vi "park.vi"() -> ()   [LabVIEW 2015]
uses:
  <vilib>/Analysis/baseanly.llb/Mean (DBL).vi
  <vilib>/Analysis/NI_AALBase.lvlib
panel:
  out "SGL error max":dbl
  out "SGL error mean":dbl format="%0.2f"
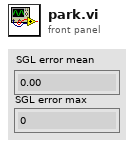
[diagram p1: front panel]
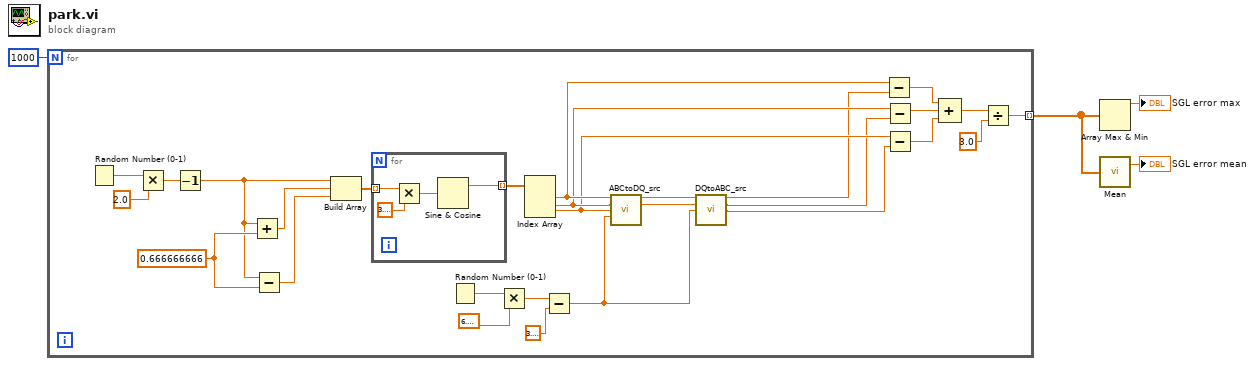
[diagram p0: block diagram]
diagram:
  n1 = for {
    N: 1000 -> [_]
    tunnel: [w19] -> w4 mode=indexing
    w30 = 0.666666666
    n2 = Random Number (0-1)() -> (number: 0 to 1=w18:dbl)
    n3 = Multiply(x=w18, y=2.0) -> (x*y=w31:dbl)
    n4 = Decrement(x=w31) -> (x-1=w25:dbl)
    n5 = Add(x=w25, y=w30) -> (x+y=w26:dbl)
    n6 = Subtract(x=w25, y=w30) -> (x-y=w27:dbl)
    n7 = Build Array(w25, w26, w27) -> (w29:dbl[])
    n8 = for {
      tunnel: w29 -> [w36] mode=indexing
      tunnel: [w34] -> w28 mode=indexing
      n9 = Multiply(x=w36, y=3.141592653589793) -> (x*y=w33:dbl)
      n10 = Sine & Cosine(0:w33) -> (1:w34:dbl)  [unwired: 1 out]
    }
    n11 = Random Number (0-1)() -> (number: 0 to 1=w17:dbl)
    n12 = Multiply(x=w17, y=6.283185307179586) -> (x*y=w12:dbl)
    n13 = Index Array(array=w28) -> (element #1=w16:dbl, element #2=w15:dbl, element #3=w14:dbl)  [unwired: 3 in]
    n14 = Subtract(x=w12, y=3.141592653589793) -> (x-y=w5:dbl)
    n15 = call "ABCtoDQ_src.vi"("A"=w16, "B"=w15, "C"=w14, "Theta"=w5) -> ("direct"=w10:sgl, "quadrature"=w9:sgl)  [unwired: 8 in, 2 out]
    n16 = call "DQtoABC_src.vi"("direct"=w10, "quadrature"=w9, "theta"=w5) -> ("A"=w8:sgl, "B"=w7:sgl, "C"=w6:sgl)  [unwired: 8 in, 2 out]
    n17 = Subtract(x=w16, y=w8) -> (x-y=w24:dbl)
    n18 = Subtract(x=w15, y=w7) -> (x-y=w23:dbl)
    n19 = Subtract(x=w14, y=w6) -> (x-y=w22:dbl)
    n20 = Compound Arithmetic op=ADD(w24, w23, w22) -> (w21:dbl)
    n21 = Divide(x=w21, y=3.0) -> (x/y=w19:dbl)
  }
  n22 = Array Max & Min(array=w4) -> (max value=→"SGL error max":dbl)  [unwired: 3 out]
  n23 = call-poly <vilib>:"Mean.vi"("X"=w4) -> ("mean"=→"SGL error mean":dbl)  [unwired: 1 out]
